vi "Read H2O Concentration DBL.vi"(8 "error in":errorcluster, 10 "Source":string, 11 "IRead Water Concentration in":refnum<class "Virtual NEO480.lvclass">) -> (0 "error out":errorcluster, 1 "Time Stamp":timestamp format="%<%x %.3X>T", 2 "H2O Concentration":dbl format="%d Vol.-%", 3 "IRead Water Concentration out":refnum<class "Virtual NEO480.lvclass">)   [LabVIEW 2024, in "Virtual NEO480.lvclass"]
uses:
  Virtual NEO480.lvclass
  Virtual NEO480.lvclass/Virtual NEO480.ctl
  Source/DBC Communicator/DBC Communicator.lvclass
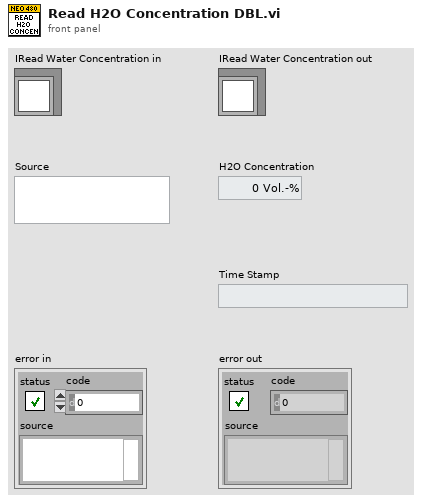
[diagram p1: front panel]
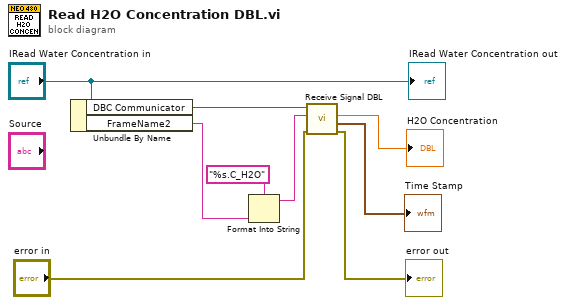
[diagram p0: block diagram]
diagram:
  n1 = Unbundle By Name("IRead Water Concentration in") -> ("DBC Communicator"=w6:refnum<class "DBC Communicator.lvclass">, "FrameName2"=w7:string)
  n2 = Format Into String(format string="%s.C_H2O", w7) -> (resulting string=w5:string)  [unwired: 2 in, 1 out]
  n3 = call "Receive Signal DBL.vi"("error in"="error in", "Signal Name"=w5, "DBC Communication in"=w6) -> ("error out"=→"error out":errorcluster, "Time Stamp"=→"Time Stamp":timestamp, "Value"=→"H2O Concentration":dbl)  [unwired: 5 in, 1 out]
  "IRead Water Concentration out" <- "IRead Water Concentration in"
